vi "encode btr.vi"(7 "triple sampling (F)":bool, 10 "clock frequency (8 MHz)":u8=8, 11 "bitrate parameters":T1) -> (3 "btr":u16 format="%x")   [LabVIEW 2024, in "atsj peakcan basic.lvlib"]
doc: "Converts <b>bitrate parameters</b> into the corresponding <b>btr</b> (Bus Timing Register) value.\n\nCopyright (c) 2025 ATSJ (www.atsj.eu)"
uses:
  bitrate parameters.ctl
  atsj peakcan basic.lvlib
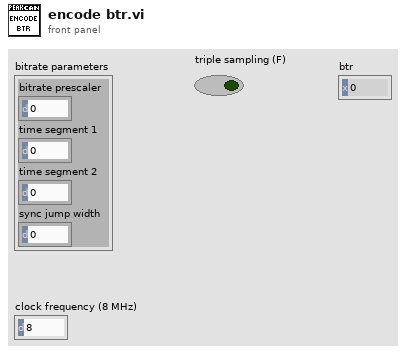
[diagram p1: front panel]
types:
  T1 = typedef "atsj peakcan basic.lvlib/bitrate parameters.ctl" = cluster{"bitrate prescaler":u16, "time segment 1":u16, "time segment 2":u16, "sync jump width":u16}
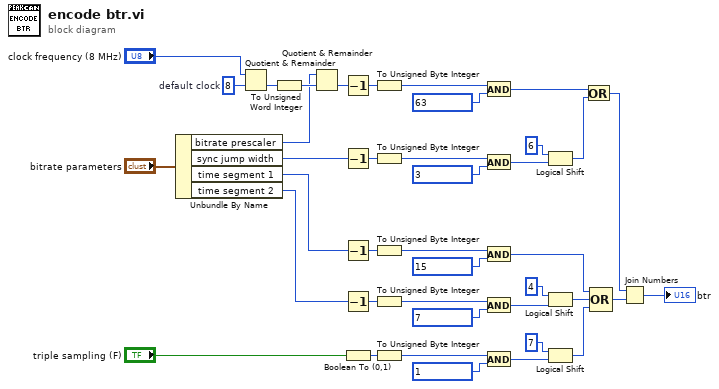
[diagram p0: block diagram]
diagram:
  w15 = u8 8  # default clock
  n1 = Unbundle By Name("bitrate parameters") -> ("bitrate prescaler"=w2:u16, "sync jump width"=w9:u16, "time segment 1"=w11:u16, "time segment 2"=w10:u16)
  n2 = Quotient & Remainder(x="clock frequency (8 MHz)", y=w15) -> (floor(x/y)=w14:u8)  [unwired: 1 out]
  n3 = To Unsigned Word Integer(number=w14) -> (unsigned 16bit integer=w7:u16)
  n4 = Quotient & Remainder(x=w2, y=w7) -> (floor(x/y)=w21:u16)  [unwired: 1 out]
  n5 = Decrement(x=w21) -> (x-1=w19:u16)
  n6 = Decrement(x=w9) -> (x-1=w1:u16)
  n7 = Decrement(x=w11) -> (x-1=w32:u16)
  n8 = Decrement(x=w10) -> (x-1=w34:u16)
  n9 = Boolean To (0,1)(Boolean="triple sampling (F)") -> (0, 1=w30:i16)
  n10 = To Unsigned Byte Integer(number=w19) -> (unsigned 8bit integer=w5:u8)
  n11 = To Unsigned Byte Integer(number=w1) -> (unsigned 8bit integer=w6:u8)
  n12 = To Unsigned Byte Integer(number=w32) -> (unsigned 8bit integer=w4:u8)
  n13 = To Unsigned Byte Integer(number=w34) -> (unsigned 8bit integer=w3:u8)
  n14 = To Unsigned Byte Integer(number=w30) -> (unsigned 8bit integer=w27:u8)
  n15 = And(x=w5, y=u8 63) -> (x .and. y?=w18:u8)
  n16 = And(x=w6, y=u8 3) -> (x .and. y?=w38:u8)
  n17 = And(x=w4, y=u8 15) -> (x .and. y?=w25:u8)
  n18 = And(x=w3, y=u8 7) -> (x .and. y?=w37:u8)
  n19 = And(x=w27, y=u8 1) -> (x .and. y?=w28:u8)
  n20 = Logical Shift(y=i16 6, x=w38) -> (x << y=w17:u8)
  n21 = Logical Shift(y=i16 4, x=w37) -> (x << y=w24:u8)
  n22 = Logical Shift(y=i16 7, x=w28) -> (x << y=w23:u8)
  n23 = Or(x=w18, y=w17) -> (x .or. y?=w16:u8)
  n24 = Compound Arithmetic op=OR(w25, w24, w23) -> (w22:u8)
  n25 = Join Numbers(hi=w16, lo=w22) -> ((hi.lo)=→"btr":u16)
